vi "Credit Update.vi"(8 "error in (no error)":errorcluster, 10 "Credit":dbl, 11 "UI Actor in":refnum<class "UI Actor.lvclass">) -> (0 "error out":errorcluster, 3 "UI Actor out":refnum<class "UI Actor.lvclass">)   [LabVIEW 2020, in "UI Actor.lvlib" / "UI Actor.lvclass"]
uses:
  UI Actor.lvclass
  UI Actor.lvclass/UI Actor.ctl
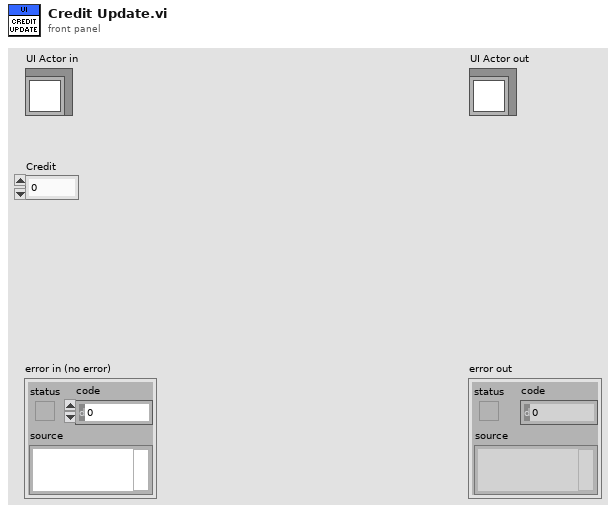
[diagram p1: front panel]
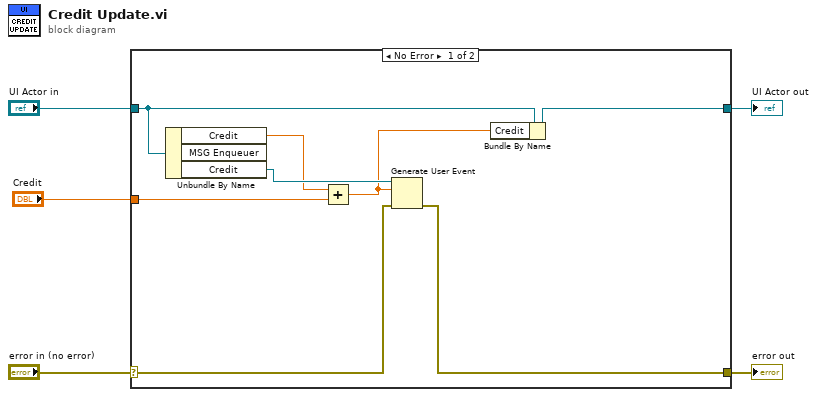
[diagram p0: block diagram]
diagram:
  n1 = case shown="No Error" "error in (no error)" {
    selector: "error in (no error)" -> [w11 w15]
    tunnel: [w8 w15] -> w4
    tunnel: [w10 w14] -> w2
    tunnel: "UI Actor in" -> [w13 w14]
    tunnel: "Credit" -> [w9 _]
    frame No Error {
      n2 = Unbundle By Name(w13) -> ("Credit"=w6:dbl, "Credit"=w12:refnum<user-event>)  [unwired: 1 out]
      n3 = Add(x=w6, y=w9) -> (x+y=w7:dbl)
      n4 = Generate User Event(user event=w12, event data cluster=w7, error in=w11) -> (error out=w8:errorcluster)  [unwired: 1 in, 1 out]
      n5 = Bundle By Name(cluster=w13, "Credit"=w7) -> (w10:refnum<class "UI Actor.lvclass">)
    }
    frame Error {
    }
  }
  "error out" <- w4
  "UI Actor out" <- w2
